vi "Error Log Example.vi"() -> ()   [LabVIEW 2017]
uses:
  Type Defs/Display Format.ctl
  Record.Error/Record.Error.lvclass
  \\192.168.1.40\Neosoft/Partage/Dossiers Personnels/BRO/DevTools_BR/wc/ErrorLog/src/Record/Record.lvclass
  Handler.UserEvent.Console/Handler.UserEvent.Console.lvclass
  \\192.168.1.40\Neosoft/Partage/Dossiers Personnels/BRO/DevTools_BR/wc/ErrorLog/src/Handler/Handler.lvclass
  Handler/Handler.lvclass
  Error Log.lvlib
panel:
  in  "Erase":bool
  in  "Display Format":T1
  in  "Show Console":bool
  in  "Error Level":T2(ring)
  in  "Error Message":string="Error log message."
  in  "Error":errorcluster={"status"=TRUE, "code"=5000, "source"="My Error Code"}
  in  "Send Error":bool
  in  "Level":T2(ring)
  in  "Name":string="User Log Example"
  in  "Show Console":bool=TRUE
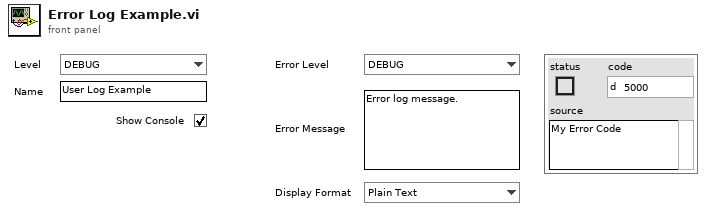
[diagram p1: front panel]
types:
  T1 = typedef "Error Log.lvlib/Display Format.ctl" = enum16{"Plain Text", "INI", "XML", "JSON"}
  T2 = enum16{"DEBUG", "INFO", "WARNING", "ERROR", "CRITICAL"}
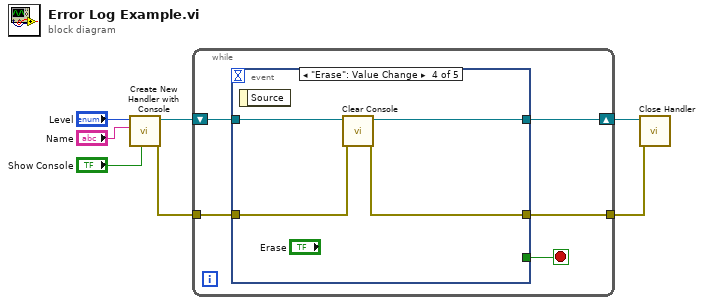
[diagram p0: block diagram]
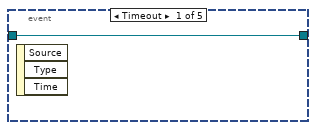
[diagram p2: hidden frame]
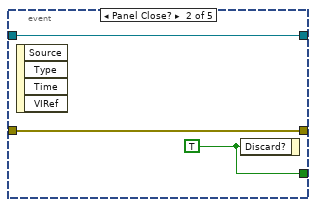
[diagram p3: hidden frame]
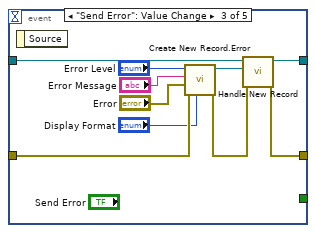
[diagram p4: hidden frame]
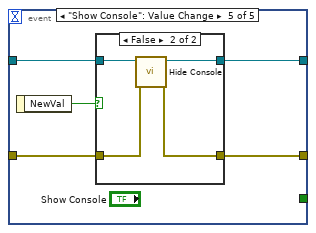
[diagram p5: hidden frame]
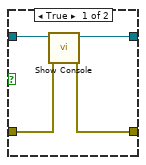
[diagram p6: hidden frame]
diagram:
  n1 = call "Create New Handler with Console.vi"("Show Console"="Show Console", "Name"="Name", "Level"="Level") -> ("error out"=w2:errorcluster, "Handler.UserEvent.Console out"=w4:refnum<class "Handler.UserEvent.Console.lvclass">)  [unwired: 7 in]
  n2 = while {
    shift-right: [w11] -> w3
    shift-left: w4 -> [w12]
    tunnel: w2 -> [w9]
    tunnel: [w8] -> w1
    stop <- w10 stop-if-true
    n3 = event shown="[3] \"Erase\": Value Change" {
      selector: _ -> [_ _ _ _ _]
      dyn-events: _ -> [_ _ _ _ _]
      timeout: _ -> [_ _ _ _ _]
      tunnel: w12 -> [w13 w16 w26 w30 w35]
      tunnel: [w13 w16 w25 w29 w34] -> w11
      tunnel: [_ w15 _ _ _] -> w10
      tunnel: w9 -> [_ w14 w19 w27 w33]
      tunnel: [_ w14 w24 w28 w32] -> w8
      event Timeout {
        n4 = event-data() -> ()  [unwired: 1 in, 3 out]
      }
      event Panel Close? {
        w15 = TRUE ("Discard?")
        n5 = event-data() -> ()  [unwired: 1 in, 4 out]
        n6 = event-data("Discard?"=w15) -> ()  [unwired: 1 in, 1 out]
      }
      event "Send Error": Value Change {
        n7 = event-data() -> ()  [unwired: 1 in, 1 out]
        n8 = call "Create New Record.Error.vi"("Display Format"="Display Format", "error in (no error)"=w19, "Error"="Error", "Message"="Error Message", "Level"="Error Level") -> ("error out"=w18:errorcluster, "Record.Error out"=w23:refnum<class "Record.Error.lvclass">)  [unwired: 5 in]
        n9 = call "Handle New Record.vi"("error in (no error)"=w18, "New Record"=w23, "Handler in"=w26) -> ("error out"=w24:errorcluster, "Handler out"=w25:refnum<class "Handler.UserEvent.Console.lvclass">)  [unwired: 7 in]
      }
      event "Erase": Value Change {
        n10 = event-data() -> ()  [unwired: 1 in, 1 out]
        n11 = call "Clear Console.vi"("error in (no error)"=w27, "Handler.UserEvent.Console in"=w30) -> ("error out"=w28:errorcluster, "Handler.UserEvent.Console out"=w29:refnum<class "Handler.UserEvent.Console.lvclass">)  [unwired: 8 in]
      }
      event "Show Console": Value Change {
        n12 = event-data() -> ("NewVal"=w31:bool)  [unwired: 1 in]
        n13 = case shown="False" w31 {
          tunnel: w35 -> [w39 w43]
          tunnel: [w38 w42] -> w34
          tunnel: w33 -> [w37 w41]
          tunnel: [w36 w40] -> w32
          frame True {
            n14 = call "Show Console.vi"("error in (no error)"=w37, "Handler.UserEvent.Console in"=w39) -> ("error out"=w36:errorcluster, "Handler.UserEvent.Console out"=w38:refnum<class "Handler.UserEvent.Console.lvclass">)  [unwired: 8 in]
          }
          frame False {
            n15 = call "Hide Console.vi"("error in (no error)"=w41, "Handler.UserEvent.Console in"=w43) -> ("error out"=w40:errorcluster, "Handler.UserEvent.Console out"=w42:refnum<class "Handler.UserEvent.Console.lvclass">)  [unwired: 8 in]
          }
        }
      }
    }
  }
  n16 = call "Close Handler.vi"("error in (no error)"=w1, "Handler in"=w3) -> ()  [unwired: 8 in, 2 out]
